vi "Get Pattern.vi"(11 "Signal Patern":string[](array[string])) -> (3 "appended array":T1[](array[typedef]))   [LabVIEW 2019, in "Day 8.lvlib"]
uses:
  Day 8.lvlib
  Controls/Digit.ctl
panel:
  out "Digit 3":string
  out "digit 5":string
  out "Digit 2":string
  out "Digit 1":string
  out "sequence":string[][](array[string])
  # "number or number of segments"
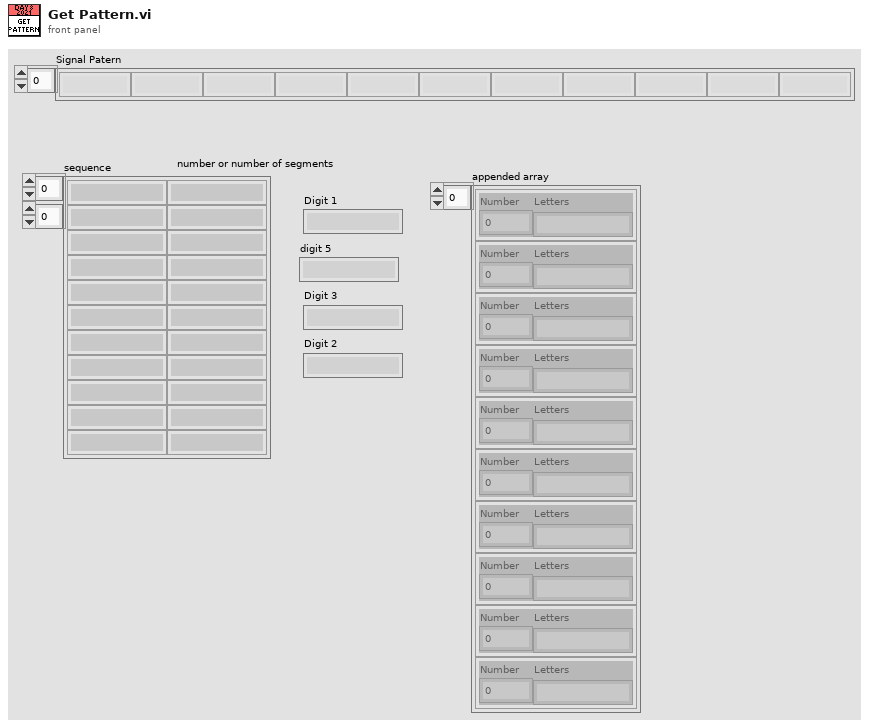
[diagram p1: front panel]
types:
  T1 = typedef "Day 8.lvlib/Digit.ctl" = cluster{"Number":u8, "Letters":string}
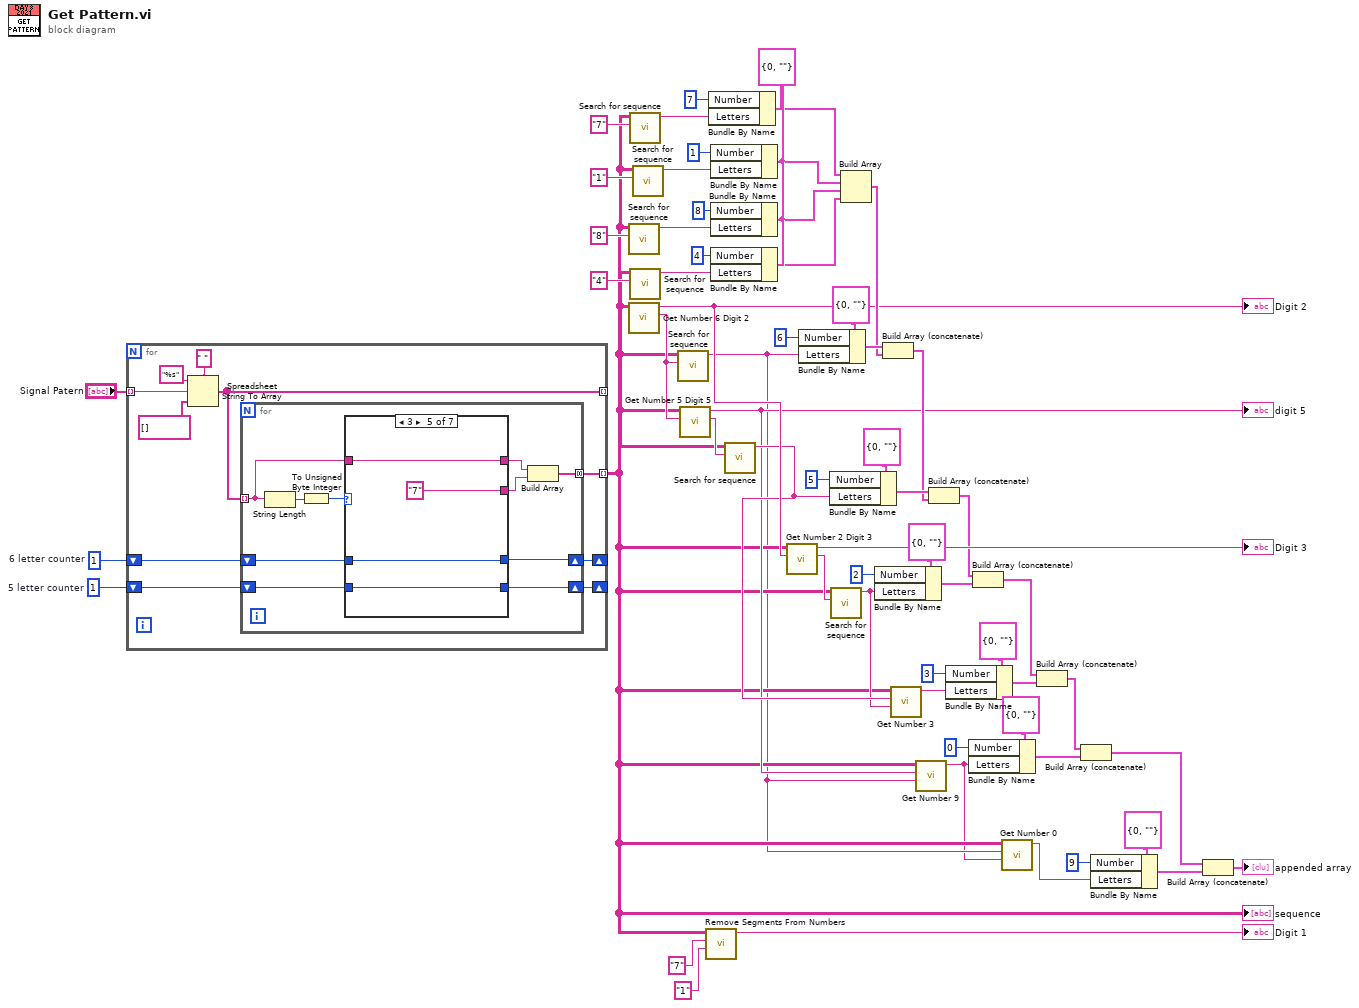
[diagram p0: block diagram]
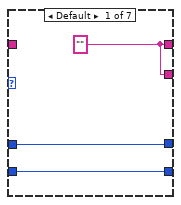
[diagram p2: hidden frame]
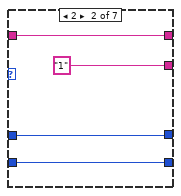
[diagram p3: hidden frame]
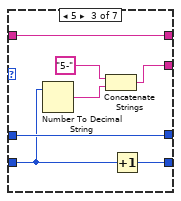
[diagram p4: hidden frame]
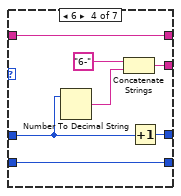
[diagram p5: hidden frame]
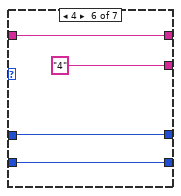
[diagram p6: hidden frame]
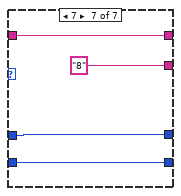
[diagram p7: hidden frame]
diagram:
  w47 = T1 {"Number"=0, "Letters"=""} ("Digit")
  w56 = 1  # 5 letter counter
  w57 = 1  # 6 letter counter
  n1 = for {
    tunnel: "Signal Patern" -> [w71] mode=indexing
    tunnel: [w67] -> _ mode=indexing
    tunnel: [w66] -> w9 mode=indexing
    shift-right: [w63] -> _
    shift-left: w57 -> [w65]
    shift-right: [w62] -> _
    shift-left: w56 -> [w64]
    n2 = Spreadsheet String To Array(delimiter (Tab)=" ", format string="%s", spreadsheet string=w71, array type (2D Dbl)=string[] []) -> (array=w67:string[])
    n3 = for {
      tunnel: w67 -> [w79] mode=indexing
      tunnel: [w76] -> w66 mode=concatenating
      shift-right: [w72] -> w63
      shift-left: w65 -> [w75]
      shift-right: [w73] -> w62
      shift-left: w64 -> [w74]
      n4 = String Length(string=w79) -> (length=w81:i32)
      n5 = To Unsigned Byte Integer(number=w81) -> (unsigned 8bit integer=w80:u8)
      n6 = case shown="3" w80 {
        tunnel: w79 -> [_ w88 w95 w102 w106 w110 w114]
        tunnel: [w84 w88 w95 w102 w106 w110 w114] -> w78
        tunnel: [w84 "1" w93 w98 "7" "4" ("format string") "8" ("format string")] -> w77
        tunnel: w75 -> [w83 w86 w91 w99 w104 w108 w112]
        tunnel: w74 -> [w82 w85 w89 w101 w103 w107 w111]
        tunnel: [w82 w85 w90 w101 w103 w107 w111] -> w73
        tunnel: [w83 w86 w91 w100 w104 w108 w112] -> w72
        frame Default {
          w84 = "" ("format string")
        }
        frame 2 {
        }
        frame 5 {
          n7 = Number To Decimal String(number=w89) -> (decimal integer string=w92:string)  [unwired: 1 in]
          n8 = Concatenate Strings("5-", w92) -> (w93:string)
          n9 = Increment(x=w89) -> (x+1=w90:i32)
        }
        frame 6 {
          n10 = Number To Decimal String(number=w99) -> (decimal integer string=w96:string)  [unwired: 1 in]
          n11 = Concatenate Strings("6-", w96) -> (w98:string)
          n12 = Increment(x=w99) -> (x+1=w100:i32)
        }
        frame 3 {
        }
        frame 4 {
        }
        frame 7 {
        }
      }
      n13 = Build Array(w78, w77) -> (w76:string[])
    }
  }
  "sequence" <- w9
  n14 = call "Search for sequence.vi"("Pattern For Number Of Letters"="8", "Array"=w9) -> ("sequence"=w46:string)  [unwired: 9 in]
  n15 = call "Get Number 6 Digit 2.vi"("Array"=w9) -> ("String"=w37:string, "Result"=w22:string)  [unwired: 9 in]
  "Digit 2" <- w22
  n16 = call "Search for sequence.vi"("Pattern For Number Of Letters"="7", "Array"=w9) -> ("sequence"=w53:string)  [unwired: 9 in]
  n17 = call "Search for sequence.vi"("Pattern For Number Of Letters"="4", "Array"=w9) -> ("sequence"=w43:string)  [unwired: 9 in]
  n18 = call "Search for sequence.vi"("Pattern For Number Of Letters"="1", "Array"=w9) -> ("sequence"=w52:string)  [unwired: 9 in]
  n19 = call "Search for sequence.vi"("Pattern For Number Of Letters"=w37, "Array"=w9) -> ("sequence"=w8:string)  [unwired: 9 in]
  n20 = call "Get Number 5 Digit 5.vi"("Pattern Number 6"=w37, "Array"=w9) -> ("Pattern number 5"=w31:string, "Digit 5"=w14:string)  [unwired: 8 in]
  "digit 5" <- w14
  n21 = call "Remove Segments From Numbers.vi"("Pattern For Letter Of Letters B"="1" ("element"), "Pattern For Number Of Letters A"="7" ("element"), "Array"=w9) -> ("Result"=→"Digit 1":string)  [unwired: 8 in]
  n22 = Bundle By Name(cluster=w47, "Number"=u8 7, "Letters"=w53) -> (w42:T1)
  n23 = Bundle By Name(cluster=w47, "Number"=u8 1, "Letters"=w52) -> (w41:T1)
  n24 = Bundle By Name(cluster=w47, "Number"=u8 8, "Letters"=w46) -> (w40:T1)
  n25 = Bundle By Name(cluster=w47, "Number"=u8 4, "Letters"=w43) -> (w39:T1)
  n26 = call "Search for sequence.vi"("Pattern For Number Of Letters"=w31, "Array"=w9) -> ("sequence"=w21:string)  [unwired: 9 in]
  n27 = call "Get Number 2 Digit 3.vi"("Digit 2"=w22, "Array"=w9) -> ("Pattern number 2"=w23:string, "Digit 3"=→"Digit 3":string)  [unwired: 8 in]
  n28 = Bundle By Name(cluster=T1 {"Number"=0, "Letters"=""} ("Digit"), "Number"=u8 6, "Letters"=w8) -> (w35:T1)
  n29 = Bundle By Name(cluster=T1 {"Number"=0, "Letters"=""} ("Digit"), "Number"=u8 5, "Letters"=w21) -> (w30:T1)
  n30 = call "Search for sequence.vi"("Pattern For Number Of Letters"=w23, "Array"=w9) -> ("sequence"=w20:string)  [unwired: 9 in]
  n31 = Build Array(w42, w41, w40, w39) -> (w34:T1[])
  n32 = Bundle By Name(cluster=T1 {"Number"=0, "Letters"=""} ("Digit"), "Number"=u8 2, "Letters"=w20) -> (w24:T1)
  n33 = Build Array (concatenate)(w35, w34) -> (w29:T1[])
  n34 = call "Get Number 3.vi"("number 2"=w20, "number 5"=w21, "Array"=w9) -> ("sequence number 3"=w18:string)  [unwired: 8 in]
  n35 = call "Get Number 9.vi"("Number 6"=w8, "Digit 5"=w14, "Array"=w9) -> ("Number 9"=w7:string)  [unwired: 8 in]
  n36 = Build Array (concatenate)(w30, w29) -> (w25:T1[])
  n37 = Bundle By Name(cluster=T1 {"Number"=0, "Letters"=""} ("Digit"), "Number"=u8 3, "Letters"=w18) -> (w15:T1)
  n38 = Bundle By Name(cluster=T1 {"Number"=0, "Letters"=""} ("Digit"), "Number"=u8 0, "Letters"=w7) -> (w10:T1)
  n39 = Build Array (concatenate)(w25, w24) -> (w16:T1[])
  n40 = call "Get Number 0.vi"("number 9"=w7, "number 6"=w8, "Array"=w9) -> ("sequence number 0"=w5:string)  [unwired: 8 in]
  n41 = Build Array (concatenate)(w16, w15) -> (w12:T1[])
  n42 = Build Array (concatenate)(w12, w10) -> (w3:T1[])
  n43 = Bundle By Name(cluster=T1 {"Number"=0, "Letters"=""} ("Digit"), "Number"=u8 9, "Letters"=w5) -> (w2:T1)
  n44 = Build Array (concatenate)(w3, w2) -> (→"appended array":T1[])
